vi "Write Label.vi"(8 "error in (no error)":errorcluster, 10 "Label":string, 11 "Pane in":refnum<class "Pane.lvclass">) -> (0 "error out":errorcluster, 3 "Pane out":refnum<class "Pane.lvclass">)   [LabVIEW 2017, in "Pane.lvclass"]
uses:
  Pane.lvclass
  Pane.lvclass/Pane.ctl
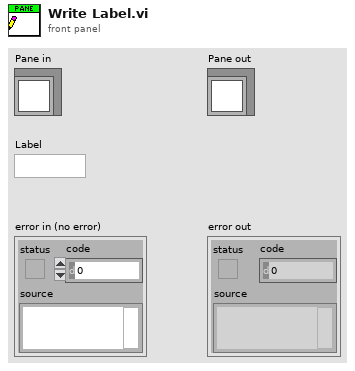
[diagram p1: front panel]
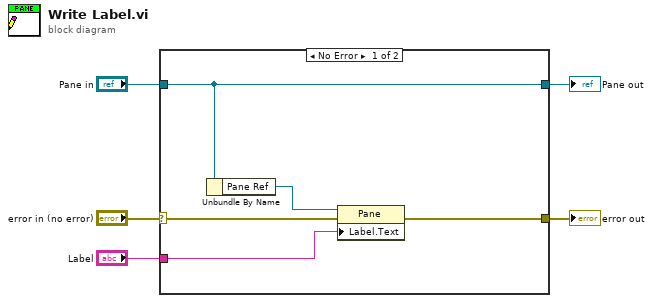
[diagram p0: block diagram]
diagram:
  n1 = case shown="No Error" "error in (no error)" {
    selector: "error in (no error)" -> [w10 w11]
    tunnel: [w9 w11] -> w4
    tunnel: [w7 w12] -> w2
    tunnel: "Pane in" -> [w7 w12]
    tunnel: "Label" -> [w8 _]
    frame No Error {
      n2 = Unbundle By Name(w7) -> ("Pane Ref"=w6:refnum<vi>)
      n3 = property class="Pane"(reference=w6, error in=w10, "Label.Text"=w8) -> (error out=w9:errorcluster)  [unwired: 1 out]
    }
    frame Error {
    }
  }
  "error out" <- w4
  "Pane out" <- w2
